vi "exersise 3-3.vi"() -> ()   [LabVIEW 2014]
panel:
  out "Temperature History":dbl(graph)
  in  "Power":bool
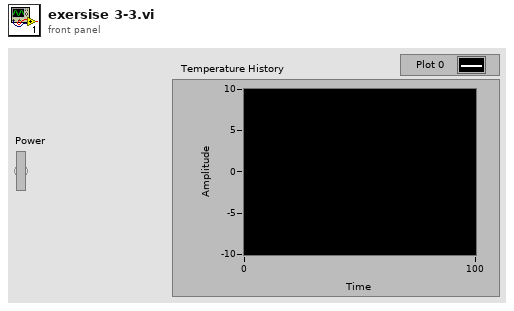
[diagram p1: front panel]
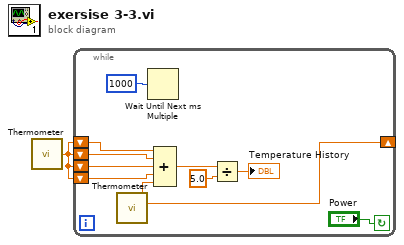
[diagram p0: block diagram]
diagram:
  n1 = call "Thermometer.vi"() -> ("Temperature"=w1:dbl)  [unwired: 1 in]
  n2 = while {
    shift-right: [w3] -> _
    shift-left: w1 -> [w9]
    shift-left: w1 -> [w6]
    shift-left: w1 -> [w8]
    shift-left: w1 -> [w7]
    stop <- "Power" continue-if-true
    n3 = call "Thermometer.vi"() -> ("Temperature"=w3:dbl)  [unwired: 1 in]
    n4 = Wait Until Next ms Multiple(millisecond multiple=1000) -> ()  [unwired: 1 out]
    n5 = Compound Arithmetic op=ADD(w9, w8, w7, w6, w3) -> (w4:dbl)
    n6 = Divide(x=w4, y=5.0) -> (x/y=→"Temperature History":dbl)
  }
